vi "ReactionWheel - autotuned.vi"() -> ()   [LabVIEW 2021]
doc: "The myRIO Project template acquires acceleration data from the onboard accelerometer and displays the changes of acceleration values in a waveform chart."
uses:
  <vilib>/Platform/TimedLoop/XDataNode/timing_clust.ctl
  <vilib>/Platform/TimedLoop/XDataNode/nitl_modes.ctl
  <vilib>/Platform/TimedLoop/XDataNode/wakeup.ctl
  <vilib>/myRIO/Instrument Drivers/Onboard IO/PWM/typedefs/PWM Reference.ctl
  <vilib>/myRIO/Common/Instrument Driver Framework/Utilities/typedefs/myRIO Generic Hardware Reference.ctl
  <vilib>/myRIO/Common/Instrument Driver Framework/Utilities/typedefs/Hardware Version Enum.ctl
  <vilib>/myRIO/Common/Instrument Driver Framework/Utilities/typedefs/myRIO v1.0 Reference.ctl
  <vilib>/myRIO/Common/Instrument Driver Framework/Utilities/typedefs/Generic FPGA Reference.ctl
  <vilib>/myRIO/Common/Instrument Driver Framework/myRIO v1.0/PWM/typedefs/PWM Channels Enum.ctl
  <vilib>/myRIO/Instrument Drivers/Onboard IO/PWM/typedefs/PWM Configuration.ctl
  <vilib>/userdefined/High Color/nirio_resource_hc.ctl
  <vilib>/myRIO/Instrument Drivers/Onboard IO/UART/typedef/VISA Configuration.ctl
  <vilib>/myRIO/Common/Instrument Driver Framework/Utilities/vis/Is FPGA Ref Available.vi
  <vilib>/myRIO/Common/Instrument Driver Framework/myRIO v1.0/PWM/vis/myRIO v1.1 Open PWM.vi
  <vilib>/myRIO/Instrument Drivers/Onboard IO/PWM/vis/Set Duty Cycle and Frequency.vi
  <vilib>/myRIO/Common/Instrument Driver Framework/Utilities/vis/Validate Channels.vi
  <vilib>/myRIO/Common/Instrument Driver Framework/myRIO v1.0/PWM/vis/myRIO v1.0 Reserve PWM.vi
  <vilib>/myRIO/Common/Instrument Driver Framework/myRIO v1.0/PWM/vis/myRIO v1.0 Build MUX Configuration PWM.vi
  <vilib>/myRIO/Common/Instrument Driver Framework/myRIO v1.0/Resource Manager/vis/myRIO v1.0 Reserve Channel List.vi
  <vilib>/myRIO/Common/Instrument Driver Framework/myRIO v1.0/Resource Manager/vis/myRIO v1.0 Create Configuration List.vi
  <vilib>/myRIO/Common/Instrument Driver Framework/myRIO v1.0/Resource Manager/vis/myRIO v1.0 Reserve Channel.vi
  <vilib>/myRIO/Common/Instrument Driver Framework/myRIO v1.0/Resource Manager/vis/myRIO v1.0 Unreserve Channel.vi
  <vilib>/myRIO/Common/Instrument Driver Framework/myRIO v1.0/Resource Manager/vis/myRIO v1.0 Build Mutex Name.vi
  <vilib>/Utility/VariantDataType/GetNumericInfo.vi
  <vilib>/Utility/error.llb/Error Cluster From Error Code.vi
  <vilib>/myRIO/Common/Instrument Driver Framework/myRIO v1.0/myRIO v1.1 Open.vi
  <vilib>/myRIO/Common/Instrument Driver Framework/Utilities/vis/IO Manager.vi
  <vilib>/myRIO/Common/Instrument Driver Framework/Utilities/vis/Configuration Manager.vi
  <vilib>/myRIO/Common/Instrument Driver Framework/myRIO v1.0/Resource Manager/vis/myRIO v1.0 Configure IO.vi
  <vilib>/myRIO/Common/Instrument Driver Framework/myRIO v1.0/myRIO v1.0 Close.vi
  <vilib>/myRIO/Common/Instrument Driver Framework/myRIO v1.0/PWM/vis/myRIO v1.0 Write PWM.vi
  <vilib>/Instr/_visa.llb/VISA Configure Serial Port (Instr).vi
  <vilib>/Platform/TimedLoop/XDataNode/XDataNode.xnode
  <vilib>/myRIO/Express VI/Onboard IO/PWM/PWM Express VI.xnode
  <vilib>/myRIO/Instrument Drivers/Onboard IO/PWM/vis/myRIO PWM Open.xnode
  <vilib>/myRIO/Express VI/Onboard IO/UART/UART Express VI.xnode
  <vilib>/myRIO/Instrument Drivers/Onboard IO/UART/UART.lvlib
  <vilib>/Platform/TimedLoop/XDataNode/XDNodeRunTimeDep.lvlib
  <vilib>/myRIO/Instrument Drivers/Onboard IO/PWM/PWM.lvlib
  <vilib>/addons/control/pid/NI_PID_autopid.lvlib
panel:
  out "UART error out 2":errorcluster
  out "PID output":dbl
  in  "minimum roll (deg)":dbl
  in  "PID\nautotune\nparameters":T1 {"control specification" min=0.0 max=2.0 step=1.0; "type of controller" min=0.0 max=2.0 step=1.0; "technique" min=0.0 max=3.0 step=1.0}
  out "Tuned PID gains":cluster{"P":dbl, "I":dbl, "D":dbl}
  out "Autotuning\ncomplete":bool
  in  "Autotune":bool
  out "Ref. error":dbl
  out "Roll reference":dbl
  out "Roll (deg)":dbl
  in  "Visualisation period (ms)":dbl=250.0
  out "PID error out":errorcluster
  in  "PID output range":cluster{"Maximum":dbl, "Minimum":dbl}={"Maximum"=100.0, "Minimum"=-100.0}
  in  "PID gains":cluster{"P":dbl, "I":dbl, "D":dbl}
  in  "UART read period (ms)":dbl=25.0
  in  "PID period (ms)":dbl=100.0
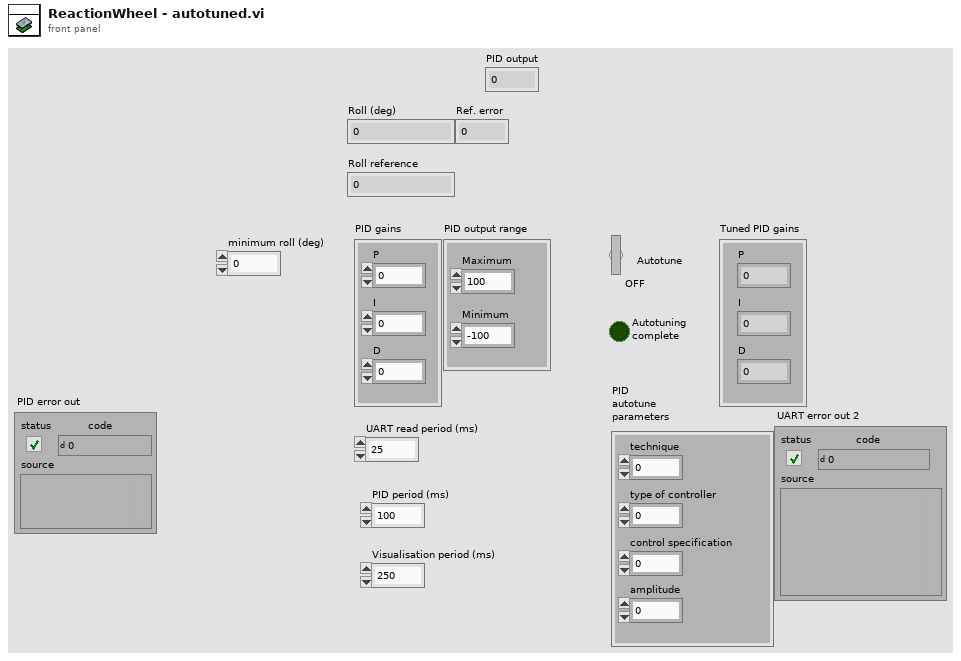
[diagram p1: front panel]
types:
  T1 = cluster{"technique":dbl, "type of controller":dbl, "control specification":dbl, "amplitude":dbl}
  T2 = cluster{"Roll (deg)":dbl, "Roll reference":dbl, "PID output":dbl}
  T3 = typedef "XDNodeRunTimeDep.lvlib/timing_clust.ctl" = cluster{"Expected End [f-1]":u64, "Actual End [f-1]":u64, "Finished Late? [f-1]":bool, "Expected End [i-1]":u64, "Actual End [i-1]":u64, "Finished Late? [i-1]":bool, "Expected Start [i]":u64, "Actual Start [i]":u64, "Expected Start [f]":u64, "Actual Start [f]":u64, "Source Name":string, "Structure Name":string, "Period":i64, "Deadline":i64, "Offset":i64, "Start":i64, "Priority":i32, "Timeout":i32, "Mode":T4, "Wakeup Reason":T5, "Error":errorcluster, "Source Type":string, "Secondary Source Type":string, "Global End Time":u64, "Global Start Time":u64, "Frame Duration":u64, "Iteration Duration":u64, "Assigned CPU":i32, "I/O Scan Engine Mode":u32}
  T4 = typedef "XDNodeRunTimeDep.lvlib/nitl_modes.ctl" = enum32{"No Change", "Process missed periods, maintain original phase", "Discard missed periods, maintain original phase", "Process missed periods, ignore original phase", "Discard missed periods, ignore original phase"}
  T5 = typedef "XDNodeRunTimeDep.lvlib/wakeup.ctl" = enum32{"Normal", "Aborted", "Asynchronous wakeup", "Timing source error", "Timed loop error", "Timeout"}
  T6 = typedef "PWM.lvlib/PWM Reference.ctl" = cluster{"myRIO Reference":T7, "PWM Channels Enum":T11, "PWM Configuration":T12}
  T7 = typedef "myRIO Generic Hardware Reference.ctl" = cluster{"myRIO Model":T8, "myRIO Hardware Reference":T9}
  T8 = typedef "Hardware Version Enum.ctl" = enum16{"Unknown", "myRIO-1900", "myRIO-1950", "roboRIO", "NI ELVIS RIO CM", "ELVIS III"}
  T9 = typedef "myRIO v1.0 Reference.ctl" = cluster{"Generic FPGA Reference":T10, "Allow multiple opens":bool}
  T10 = typedef "Generic FPGA Reference.ctl" = refnum<k20>
  T11 = typedef "PWM Channels Enum.ctl" = enum16{"Not Connected", "C/PWM0", "C/PWM1", "A/PWM0", "A/PWM1", "A/PWM2", "A/PWM3", "A/PWM4", "A/PWM5", "A/PWM6", "A/PWM7", "A/PWM8", "A/PWM9", "A/PWM10", "A/PWM11", "A/PWM12", "A/PWM13", "A/PWM14", "A/PWM15", "A/PWM16", "A/PWM17", "A/PWM18", "A/PWM19", "B/PWM0", "B/PWM1", "B/PWM2", "B/PWM3", "B/PWM4", "B/PWM5", "B/PWM6", "B/PWM7", "B/PWM8", "B/PWM9", "B/PWM10", "B/PWM11", "B/PWM12", "B/PWM13", "B/PWM14", "B/PWM15", "B/PWM16", "B/PWM17", "B/PWM18", "B/PWM19", "PWM/PWM0", "PWM/PWM1", "PWM/PWM2", "PWM/PWM3", "PWM/PWM4", "PWM/PWM5", "PWM/PWM6", "PWM/PWM7", "PWM/PWM8", "PWM/PWM9"}
  T12 = typedef "PWM.lvlib/PWM Configuration.ctl" = cluster{"Frequency":dbl, "Duty Cycle":dbl}
  T13 = typedef "nirio_resource_hc.ctl" = tag
  T14 = cluster{"proportional gain (Kc)":dbl, "integral time (Ti, min)":dbl, "derivative time (Td, min)":dbl}
  T15 = typedef "UART.lvlib/VISA Configuration.ctl" = cluster{"baud rate (9600)":u32, "data bits (8)":u16, "parity (0:none)":enum16{"None", "Odd", "Even", "Mark", "Space"}, "stop bits (10: 1 bit)":u16, "flow control (0:none)":u16, "termination char\n(0xA = '\\n' = LF) ":u8, "Enable Termination\nChar (T)":bool, "timeout (10sec)":u32}
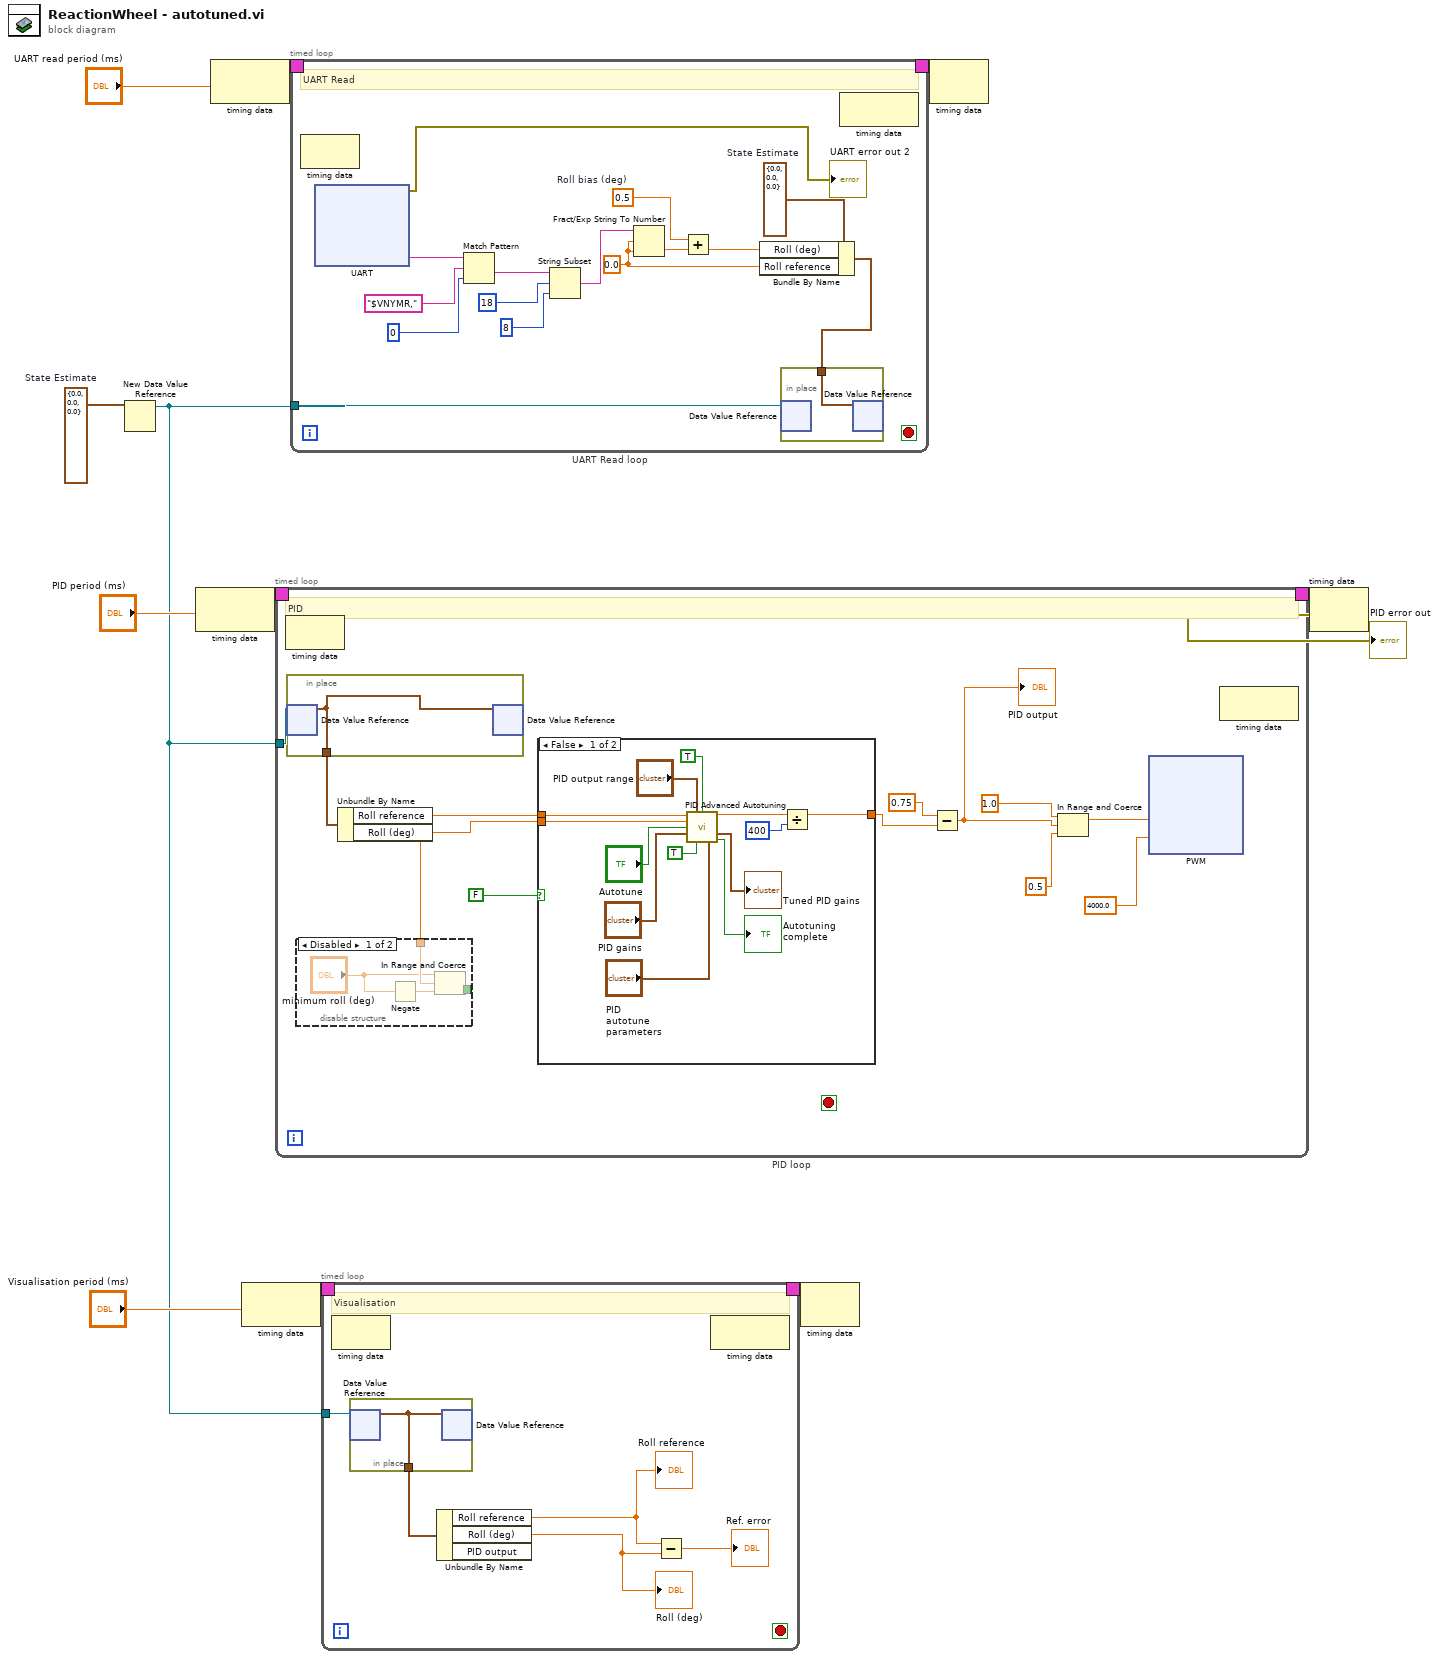
[diagram p0: block diagram]
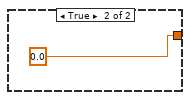
[diagram p3: hidden frame]
diagram:
  w6 = T2 {"Roll (deg)"=0.0, "Roll reference"=0.0, "PID output"=0.0}  # State Estimate
  n1 = New Data Value Reference(data value=w6) -> (data value reference=w1:refnum<data-value>)  [unwired: 1 in, 1 out]
  n2 = node-c288("PID period (ms)") -> (w10:T3)
  n3 = node-c288("UART read period (ms)") -> (w12:T3)
  n4 = node-c288("Visualisation period (ms)") -> (w4:T3)
  n5 = timed-loop "PID loop" {
    timing: w10 -> [_]
    timing-out: [_] -> w9
    tunnel: w1 -> [w23]
    stop <- _ stop-if-true
    # "PID"
    n6 = node-c288() -> ()  [unwired: 1 in, 1 out]
    n7 = in-place {
      in-place-border: [w43] -> w22
      n8 = in-place-dvr #1(w23) -> (w43:T2)  [unwired: 1 out]
      n9 = in-place-dvr #1(w43) -> ()  [unwired: 2 out]
    }
    n10 = Unbundle By Name(w22) -> ("Roll reference"=w21:dbl, "Roll (deg)"=w20:dbl)
    n11 = disable-structure shown="Disabled" {
      disable-tunnel: [w28 _] -> _
      disable-tunnel: w20 -> [w27 _]
      frame Disabled {
        n12 = Negate(x="minimum roll (deg)") -> (-x=w25:dbl)
        n13 = In Range and Coerce(upper limit="minimum roll (deg)", x=w27, lower limit=w25) -> (In Range?=w28:bool)  [unwired: 1 out]
      }
      frame Enabled {
      }
    }
    n14 = case shown="False" FALSE {
      tunnel: w21 -> [w40 _]
      tunnel: w20 -> [w31 _]
      tunnel: [w30 0.0] -> w15
      frame False {
        n15 = call <vilib>:"PID Advanced Autotuning.vi"("setpoint"=w40, "output range"="PID output range", "auto? (F)"=TRUE, "process variable"=w31, "autotune? (F)"="Autotune", "PID gains"="PID gains", "reinitialize? (F)"=TRUE, "autotuning parameters"="PID\nautotune\nparameters") -> ("output"=w38:dbl, "tuned PID gains"=→"Tuned PID gains":T14, "tuning completed?"=→"Autotuning\ncomplete":bool)  [unwired: 5 in]
        n16 = Divide(x=w38, y=400) -> (x/y=w30:dbl)
      }
      frame True {
      }
    }
    n17 = Subtract(x=0.75, y=w15) -> (x-y=w18:dbl)
    "PID output" <- w18
    n18 = In Range and Coerce(upper limit=1.0 ("Max PWM"), x=w18, lower limit=0.5 ("Min PWM")) -> (coerced(x)=w19:dbl)  [unwired: 1 out]
    n19 = xnode "PWM"("Duty Cycle"=w19, "Frequency [Hz]"=4000.0 ("PWMfrekvens")) -> ()  [unwired: 1 in, 1 out]
    n20 = node-c288() -> ()  [unwired: 1 in, 1 out]
  }
  n21 = timed-loop "UART Read loop" {
    timing: w12 -> [_]
    timing-out: [_] -> w11
    tunnel: w1 -> [w88]
    stop <- _ stop-if-true
    w82 = 0.5  # Roll bias (deg)
    w86 = T2 {"Roll (deg)"=0.0, "Roll reference"=0.0, "PID output"=0.0}  # State Estimate
    w84 = 0.0
    # "UART Read"
    n22 = node-c288() -> ()  [unwired: 1 in, 1 out]
    n23 = xnode "UART"() -> ("Characters Read"=w95:string, "error out"=→"UART error out 2":errorcluster)  [unwired: 1 in]
    n24 = Match Pattern(string=w95, regular expression="$VNYMR,", offset (0)=0) -> (after substring=w94:string)  [unwired: 3 out]
    n25 = String Subset(string=w94, offset (0)=18, length (rest)=8) -> (substring=w89:string)
    n26 = Fract/Exp String To Number(string=w89, offset=w84, default (0 dbl)=w84) -> (number=w85:dbl)  [unwired: 1 in, 1 out]
    n27 = Add(x=w82, y=w85) -> (x+y=w83:dbl)
    n28 = Bundle By Name(cluster=w86, "Roll (deg)"=w83, "Roll reference"=w84) -> (w87:T2)
    n29 = in-place {
      in-place-border: w87 -> [w96]
      n30 = in-place-dvr #2(w88) -> ()  [unwired: 2 out]
      n31 = in-place-dvr #2(w96) -> ()  [unwired: 2 out]
    }
    n32 = node-c288() -> ()  [unwired: 1 in, 1 out]
  }
  n33 = timed-loop {
    timing: w4 -> [_]
    timing-out: [_] -> w3
    tunnel: w1 -> [w120]
    stop <- _ stop-if-true
    # "Visualisation"
    n34 = node-c288() -> ()  [unwired: 1 in, 1 out]
    n35 = in-place {
      in-place-border: [w121] -> w119
      n36 = in-place-dvr #3(w120) -> (w121:T2)  [unwired: 1 out]
      n37 = in-place-dvr #3(w121) -> ()  [unwired: 2 out]
    }
    n38 = Unbundle By Name(w119) -> ("Roll reference"=w117:dbl, "Roll (deg)"=w116:dbl)  [unwired: 1 out]
    "Roll (deg)" <- w116
    "Roll reference" <- w117
    n39 = Subtract(x=w117, y=w116) -> (x-y=→"Ref. error":dbl)
    n40 = node-c288() -> ()  [unwired: 1 in, 1 out]
  }
  n41 = node-c288(w3) -> ()  [unwired: 1 out]
  n42 = node-c288(w11) -> ()  [unwired: 1 out]
  n43 = node-c288(w9) -> (→"PID error out":errorcluster)
